vi "Pre Launch Init.vi"(11 "BlinkyLightModel In":refnum<class "BlinkyLightModel.lvclass">) -> (0 "error out":errorcluster, 3 "BlinkyLightModel Out":refnum<class "BlinkyLightModel.lvclass">)   [LabVIEW 2017, in "BlinkyLightModel.lvlib" / "BlinkyLightModel.lvclass"]
doc: "(<B>Filename</B>: Actor Framework.lvlib:Actor.lvclass:Pre Launch Init.vi)\n\nDefines behavior that occurs after the Launch Nested Actor method is invoked but before the actor's Actor Core method begins running.\n\nBy default, this method does nothing. A descendant class may override it to define behavior.MVA Framework 1.7.0.33\nEthan Stern - Composed Systems\nCopyright (c) 2018, Composed Systems"
uses:
  BlinkyLightModel.lvclass
  C:/Program Files/National Instruments/LabVIEW 2017/vi.lib/ActorFramework/Actor/Actor.lvclass
  <vilib>/ActorFramework/Actor/Actor.lvclass/Actor.ctl
  <vilib>/ActorFramework/Message Enqueuer/Message Enqueuer.lvclass/Message Enqueuer.ctl
  BlinkyLightModel.lvclass/BlinkyLightModel.ctl
  <vilib>/ActorFramework/Message Enqueuer/Init from Existing Queue.vi
  <vilib>/ActorFramework/Message Enqueuer/Enqueue.vi
  BlinkyLightModel Messages/Blink Lights Msg/Blink Lights Msg.lvclass
  C:/Program Files/National Instruments/LabVIEW 2017/vi.lib/ActorFramework/Message/Message.lvclass
  <vilib>/ActorFramework/Message Priority Queue/Priority Enqueue.vi
  mva-core/Source/IModel/IModel/IModel.lvclass
  <vilib>/ActorFramework/Message Enqueuer/Message Enqueuer.lvclass
  <vilib>/ActorFramework/Actor/Actor.lvclass
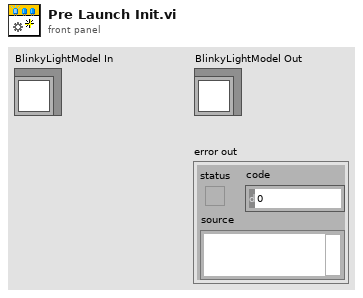
[diagram p1: front panel]
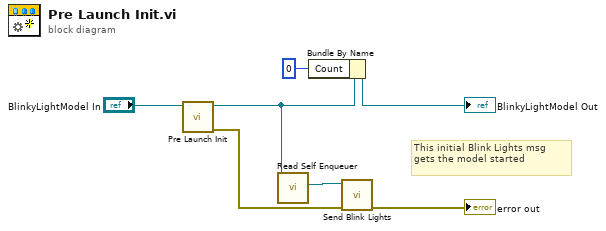
[diagram p0: block diagram]
diagram:
  # "This initial Blink Lights msg\ngets the model started"
  n1 = call-parent "Pre Launch Init.vi"("IModel in"="BlinkyLightModel In") -> ("error out"=w4:errorcluster, "IModel out"=w6:refnum<class "BlinkyLightModel.lvclass">)  [unwired: 9 in]
  n2 = call <vilib>:"Read Self Enqueuer.vi"("Actor"=w6) -> ("Self Enqueuer"=w5:refnum<class "Message Enqueuer.lvclass">)  [unwired: 10 in]
  n3 = Bundle By Name(cluster=w6, "Count"=0 ("Numbers Generated")) -> (→"BlinkyLightModel Out":refnum<class "BlinkyLightModel.lvclass">)
  n4 = call "Send Blink Lights.vi"("error in (no error)"=w4, "Message Enqueuer"=w5) -> ("error out"=→"error out":errorcluster)  [unwired: 8 in, 1 out]
